vi "Water level detecter1.vi"() -> ()   [LabVIEW 2021]
panel:
  in  "stop":bool
  out "Middle Water Level":bool
  out "Low Water Level":bool
  out "High Water Level":bool
  in  "Slide":dbl(slide) scale=0.0..10.0
  out "Tank":dbl(slide) scale=0.0..10.0
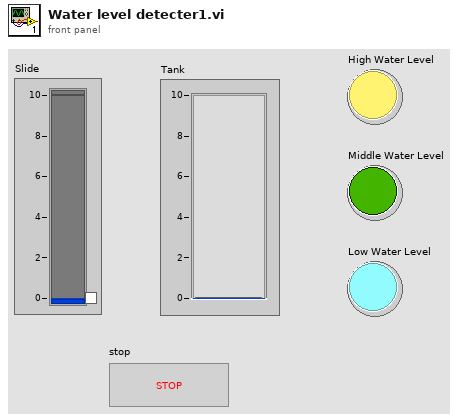
[diagram p1: front panel]
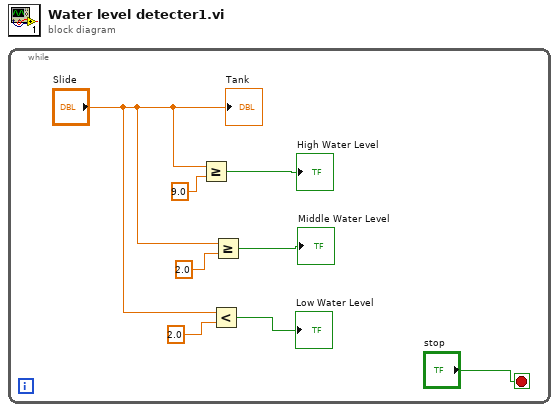
[diagram p0: block diagram]
diagram:
  n1 = while {
    stop <- "stop" stop-if-true
    n2 = Greater Or Equal?(x="Slide", y=9.0) -> (x >= y?=→"High Water Level":bool)
    n3 = Less?(x="Slide", y=2.0) -> (x < y?=→"Low Water Level":bool)
    n4 = Greater Or Equal?(x="Slide", y=2.0) -> (x >= y?=→"Middle Water Level":bool)
    "Tank" <- "Slide"
  }
